vi "TCP Communicator - Active.vi"() -> ()   [LabVIEW 2019]
doc: "Demonstrates how to display an interactive send and receive message dialog for communication between TCP connections. It establishes a connection on the machine listed and the port specified. It then waits for you to input data into the Input Line string control and hit enter. Once you hit enter, the string you typed is sent to the port and passed to the TCP Communicator - Passive.vi where it is displayed on a string indicator.\n\nThe key difference between the Active and Passive VIs is that the Active VI establishes a connection, while the Passive VI waits for a connection to be established.\n\n<B>Note:</B> Requires the TCP Communicator - Passive.vi."
panel:
  in  "Port":u16=6342
  in  "Machine":string="localhost"
  out "Their Response:":string
  in  "stop":bool
  out "You Typed:":string
  in  "Input Line":string
  # "Instructions:\n1. Open the TCP\n    Communicator - Passive.vi\n    and run it first.\n2. Run TCP Communicator - \n    Active.vi second.\n3.Type into the Input Line\n    String Control and then\n    hit Enter.\n4. Type into the Input Line\n    of the other VI and then\n    hit Enter.\n5. Press Stop to end session."
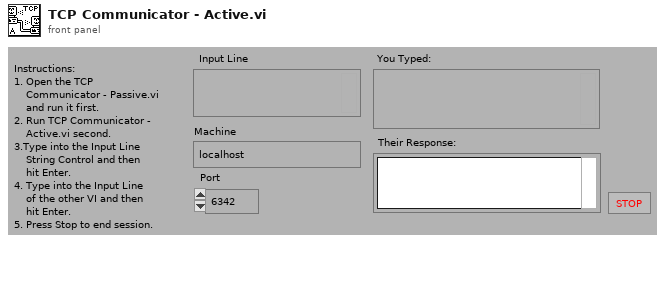
[diagram p1: front panel]
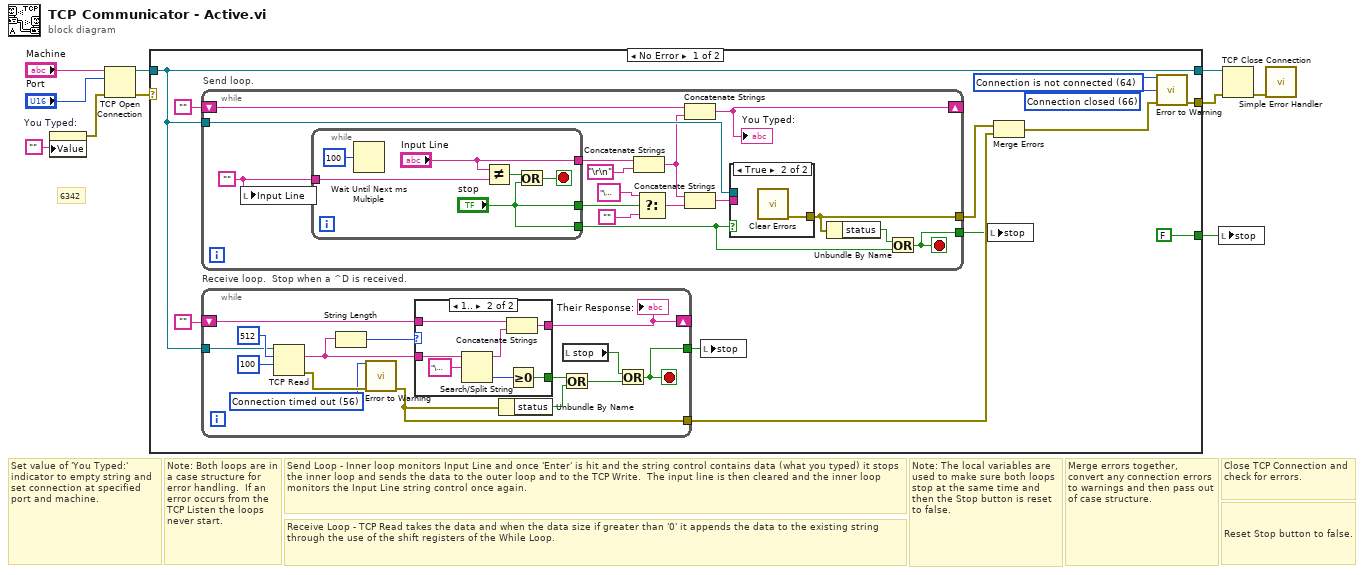
[diagram p0: block diagram]
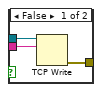
[diagram p2: hidden frame]
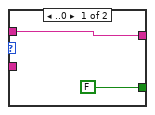
[diagram p3: hidden frame]
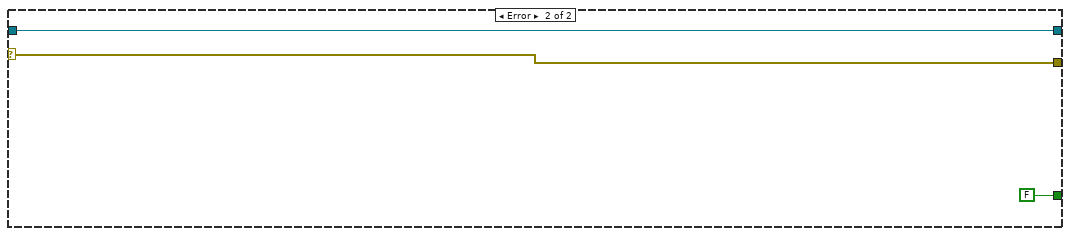
[diagram p4: hidden frame]
diagram:
  # "6342"
  # "Set value of 'You Typed:' indicator to empty string and set connection at specified port and machine."
  # "Send Loop - Inner loop monitors Input Line and once 'Enter' is hit and the string control contains data (what you typed) it stops the inner loop and sends the data to the outer loop and to the TCP Write.  The input line is then cleared and the inner loop monitors the Input Line string control once again."
  # "Receive Loop - TCP Read takes the data and when the data size if greater than '0' it appends the data to the existing string through the use of the shift registers of the While Loop."
  # "Note: The local variables are used to make sure both loops stop at the same time and then the Stop button is reset to false."
  # "Merge errors together, convert any connection errors to warnings and then pass out of case structure."
  # "Note: Both loops are in a case structure for error handling.  If an error occurs from the TCP Listen the loops never start."
  # "Close TCP Connection and check for errors."
  # "Reset Stop button to false."
  n1 = property on="You Typed:" class="Str"("Value"="") -> (error out=w5:errorcluster)  [unwired: 2 in, 1 out]
  n2 = TCP Open Connection(address="Machine", remote port or service name="Port", error in (no error)=w5) -> (connection ID=w7:refnum<k5>, error out=w8:errorcluster)  [unwired: 2 in]
  n3 = case shown="No Error" w8 {
    selector: w8 -> [_ w74]
    tunnel: [w14 w74] -> w3
    tunnel: w7 -> [w20 w75]
    tunnel: [w20 w75] -> w4
    tunnel: [FALSE FALSE] -> w1
    frame No Error {
      w15 = 66 items=["No Error", "Argument Error", "Memory Full", "Out of Zone", "End of File", "File Already Open", "Generic File IO Error", "File Not Found", "File Permission Error", "Disk Full", "Duplicate Path", "Too Many Files Open", "Not Enabled", "Resource File Not Found", "Cannot Add Resource", "Resource Not Found", "Image Not Found", "Image Memory Error", "Pen Does Not Exist", "Config Bad Type", "Config Token Not Found", "Config Parse Error", "Config Memory Error", "Bad External Code Format", "Bad External Code Offset", "External Code Not Present", "Null Window", "Destroy Window Mixup", "Null Menu", "Print Aborted", "Bad Print Record", "Print Driver Error", "Windows Error During Print", "Memory Error During Print", "Print Dialog Error", "Generic Print Error", "Invalid Device Refnum", "Device Not Found", "Device Parameter Error", "Device Unit Error", "Can't Open Device", "Device Call Aborted", "Generic Error", "Cancelled By User", "Object ID Too Low", "Object ID Too High", "Object Not In Heap", "Unknown Heap", "Bad DefProc ID", "DefProc Not In Table", "Message Out Of Range", "Null Method", "Unknown Message", "Manager Call Not Supported", "Bad address", "Connection In progress", "Connection timed out", "Connection is already in progress", "Network attribute not supported", "Network error", "Address in use", "System out of memory", "Connection aborted", "Connection refused", "Connection is not connected", "Connection is already connected", "Connection closed", "Initialize error (interapplication manager)", "Bad occurrence", "Wait on unbound occurrence handler", "Occurrence queue overflow", "Bad path", "Semaphore not signaled", "Unrecognized type (interapplication manager)"] ("3rd Error to Convert")
      w16 = 64 items=["No Error", "Argument Error", "Memory Full", "Out of Zone", "End of File", "File Already Open", "Generic File IO Error", "File Not Found", "File Permission Error", "Disk Full", "Duplicate Path", "Too Many Files Open", "Not Enabled", "Resource File Not Found", "Cannot Add Resource", "Resource Not Found", "Image Not Found", "Image Memory Error", "Pen Does Not Exist", "Config Bad Type", "Config Token Not Found", "Config Parse Error", "Config Memory Error", "Bad External Code Format", "Bad External Code Offset", "External Code Not Present", "Null Window", "Destroy Window Mixup", "Null Menu", "Print Aborted", "Bad Print Record", "Print Driver Error", "Windows Error During Print", "Memory Error During Print", "Print Dialog Error", "Generic Print Error", "Invalid Device Refnum", "Device Not Found", "Device Parameter Error", "Device Unit Error", "Can't Open Device", "Device Call Aborted", "Generic Error", "Cancelled By User", "Object ID Too Low", "Object ID Too High", "Object Not In Heap", "Unknown Heap", "Bad DefProc ID", "DefProc Not In Table", "Message Out Of Range", "Null Method", "Unknown Message", "Manager Call Not Supported", "Bad address", "Connection In progress", "Connection timed out", "Connection is already in progress", "Network attribute not supported", "Network error", "Address in use", "System out of memory", "Connection aborted", "Connection refused", "Connection is not connected", "Connection is already connected", "Connection closed", "Initialize error (interapplication manager)", "Bad occurrence", "Wait on unbound occurrence handler", "Occurrence queue overflow", "Bad path", "Semaphore not signaled", "Unrecognized type (interapplication manager)"] ("1st Error to Convert")
      n4 = while "Send loop." {
        tunnel: w20 -> [w35]
        tunnel: [w37] -> w13
        tunnel: [w26] -> w18
        shift-left: "" -> [w38]
        shift-right: [w36] -> _
        stop <- w37 stop-if-true
        w24 = ""
        n5 = local write "Input Line"(w24) -> ()
        n6 = while {
          tunnel: ["stop"] -> w31
          tunnel: ["stop"] -> w23
          tunnel: ["Input Line"] -> w32
          tunnel: w24 -> [w40]
          stop <- w42 stop-if-true
          n7 = Wait Until Next ms Multiple(millisecond multiple=u32 100) -> ()  [unwired: 1 out]
          n8 = Not Equal?(x="Input Line", y=w40) -> (x != y?=w43:bool)
          n9 = Or(x=w43, y="stop") -> (x .or. y?=w42:bool)
        }
        n10 = Concatenate Strings(w32, "\r\n") -> (w28:string)
        n11 = Select(t="\u0004", s=w31, f="") -> (s? t:f=w33:string)
        n12 = Concatenate Strings(w38, w28) -> (w36:string)
        "You Typed:" <- w36
        n13 = Concatenate Strings(w28, w33) -> (w27:string)
        n14 = case shown="True" w23 {
          tunnel: w27 -> [w47 _]
          tunnel: [w46 w48] -> w26
          tunnel: w35 -> [w45 _]
          frame False {
            n15 = TCP Write(connection ID=w45, data in=w47) -> (error out=w46:errorcluster)  [unwired: 2 in, 2 out]
          }
          frame True {
            n16 = call <vilib>:"Clear Errors.vi"() -> ("error out"=w48:errorcluster)  [unwired: 6 in, 1 out]
          }
        }
        n17 = Unbundle By Name(w26) -> ("status"=w25:bool)
        n18 = Or(x=w25, y=w23) -> (x .or. y?=w37:bool)
      }
      n19 = while "Receive loop.  Stop when a ^D is received." {
        shift-left: "" -> [w60]
        shift-right: [w59] -> _
        tunnel: [w53] -> w19
        tunnel: w20 -> [w61]
        tunnel: [w49] -> w12
        stop <- w49 stop-if-true
        w54 = 56 items=["No Error", "Argument Error", "Memory Full", "Out of Zone", "End of File", "File Already Open", "Generic File IO Error", "File Not Found", "File Permission Error", "Disk Full", "Duplicate Path", "Too Many Files Open", "Not Enabled", "Resource File Not Found", "Cannot Add Resource", "Resource Not Found", "Image Not Found", "Image Memory Error", "Pen Does Not Exist", "Config Bad Type", "Config Token Not Found", "Config Parse Error", "Config Memory Error", "Bad External Code Format", "Bad External Code Offset", "External Code Not Present", "Null Window", "Destroy Window Mixup", "Null Menu", "Print Aborted", "Bad Print Record", "Print Driver Error", "Windows Error During Print", "Memory Error During Print", "Print Dialog Error", "Generic Print Error", "Invalid Device Refnum", "Device Not Found", "Device Parameter Error", "Device Unit Error", "Can't Open Device", "Device Call Aborted", "Generic Error", "Cancelled By User", "Object ID Too Low", "Object ID Too High", "Object Not In Heap", "Unknown Heap", "Bad DefProc ID", "DefProc Not In Table", "Message Out Of Range", "Null Method", "Unknown Message", "Manager Call Not Supported", "Bad address", "Connection In progress", "Connection timed out", "Connection is already in progress", "Network attribute not supported", "Network error", "Address in use", "System out of memory", "Connection aborted", "Connection refused", "Connection is not connected", "Connection is already connected", "Connection closed", "Initialize error (interapplication manager)", "Bad occurrence", "Wait on unbound occurrence handler", "Occurrence queue overflow", "Bad path", "Semaphore not signaled", "Unrecognized type (interapplication manager)"] ("1st Error to Convert")
        n20 = TCP Read(connection ID=w61, bytes to read=512, 9:100) -> (data out=w58:string, error out=w55:errorcluster)  [unwired: 2 in, 1 out]
        n21 = String Length(string=w58) -> (length=w63:i32)
        n22 = call <vilib>:"Error to Warning.vi"("1st Error to Convert"=w54, "error in"=w55) -> ("warning out"=w53:errorcluster)  [unwired: 13 in]
        n23 = case shown="1.." w63 {
          tunnel: w58 -> [_ w69]
          tunnel: w60 -> [w65 w72]
          tunnel: [w65 w71] -> w59
          tunnel: [FALSE w66] -> w57
          frame ..0 {
          }
          frame 1.. {
            n24 = Search/Split String(string=w69, search string/char (-)="\u0004") -> (substring before match=w68:string, offset of match=w67:i32)  [unwired: 1 in, 1 out]
            n25 = Concatenate Strings(w72, w68) -> (w71:string)
            n26 = Greater Or Equal To 0?(x=w67) -> (x >= 0?=w66:bool)
          }
        }
        "Their Response:" <- w59
        n27 = Unbundle By Name(w53) -> ("status"=w52:bool)
        n28 = Or(x=w57, y=w52) -> (x .or. y?=w50:bool)
        n29 = local read "stop"() -> (w51:bool)
        n30 = Or(x=w51, y=w50) -> (x .or. y?=w49:bool)
      }
      n31 = local write "stop"(w12) -> ()
      n32 = local write "stop"(w13) -> ()
      n33 = Merge Errors(w18, w19) -> (w17:errorcluster)
      n34 = call <vilib>:"Error to Warning.vi"("1st Error to Convert"=w16, "3rd Error to Convert"=w15, "error in"=w17) -> ("warning out"=w14:errorcluster)  [unwired: 12 in]
    }
    frame Error {
    }
  }
  n35 = local write "stop"(w1) -> ()
  n36 = TCP Close Connection(connection ID=w4, error in (no error)=w3) -> (error out=w2:errorcluster)  [unwired: 1 in, 1 out]
  n37 = call <vilib>:"Simple Error Handler.vi"("error in (no error)"=w2) -> ()  [unwired: 4 in, 5 out]
